vi "SetCal.vi"(8 "Sleep":u32=200, 9 "DoIt":bool=TRUE, 10 "R":dbl[](array[numeric])) -> (0 "Sleep":u32)   [LabVIEW 2025]
uses:
  Globals.vi
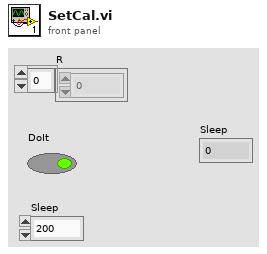
[diagram p1: front panel]
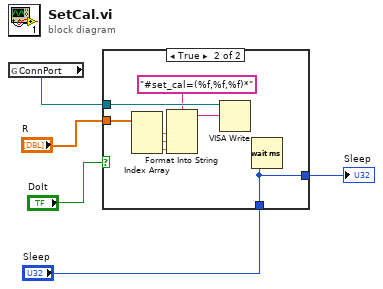
[diagram p0: block diagram]
diagram:
  n1 = global read "Globals.vi" "ConnPort"() -> (w1:refnum<visa-resource-name>)
  n2 = case shown="True" "DoIt" {
    tunnel: w1 -> [_ w14]
    tunnel: "R" -> [_ w8]
    tunnel: "Sleep" -> [w6 w7]
    tunnel: [w6 w7] -> w2
    frame False {
    }
    frame True {
      n3 = Index Array(array=w8) -> (element #1=w11:dbl, element #2=w12:dbl, element #3=w13:dbl)  [unwired: 3 in]
      n4 = Format Into String(format string="#set_cal=(%f,%f,%f)*", w11, w12, w13) -> (resulting string=w10:string)  [unwired: 2 in, 1 out]
      n5 = VISA Write(VISA resource name=w14, write buffer=w10) -> ()  [unwired: 1 in, 3 out]
      n6 = Wait (ms)(milliseconds to wait=w7) -> ()  [unwired: 1 out]
    }
  }
  "Sleep" <- w2
